vi "doAction.vi"(8 "error in (no error)":errorcluster, 11 "Stop in":refnum<class "Stop.lvclass">) -> (0 "error out":errorcluster, 3 "Stop out":refnum<class "Stop.lvclass">)   [LabVIEW 2018, in "Stop.lvclass"]
uses:
  Stop.lvclass
  State/State.lvclass
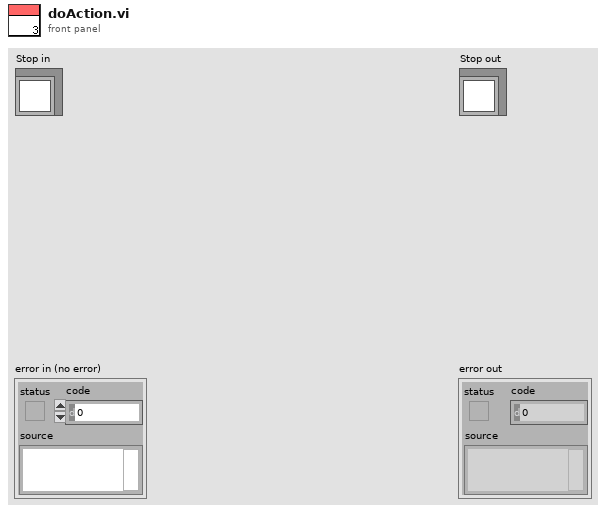
[diagram p1: front panel]
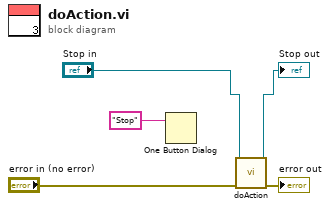
[diagram p0: block diagram]
diagram:
  n1 = One Button Dialog(message="Stop") -> ()  [unwired: 1 in, 1 out]
  n2 = call-parent "doAction.vi"("error in (no error)"="error in (no error)", "State in"="Stop in") -> ("error out"=→"error out":errorcluster, "State out"=→"Stop out":refnum<class "Stop.lvclass">)  [unwired: 8 in]
